vi "NP_IOW_LaunchTheServer.vi"(5 "error in (no error)":errorcluster) -> (19 "error out":errorcluster)   [LabVIEW 2010]
uses:
  <vilib>/registry/registry.llb/Registry View.ctl
  <vilib>/registry/registry.llb/Registry SAM.ctl
  <vilib>/registry/registry.llb/Registry RtKey.ctl
  <vilib>/registry/registry.llb/Read Registry Value Simple STR.vi
panel:
  out "NSTRUCT Instrument Manager path":string
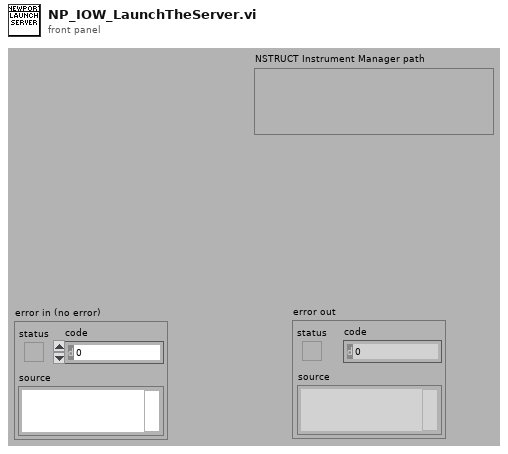
[diagram p1: front panel]
types:
  T1 = typedef "Registry SAM.ctl" = enum32{"KEY_QUERY_VALUE", "KEY_SET_VALUE", "KEY_CREATE_SUB_KEY", "KEY_ENUMERATE_SUB_KEYS", "KEY_NOTIFY", "KEY_CREATE_LINK", "KEY_READ", "KEY_WRITE", "KEY_ALL_ACCESS", "KEY_READ | KEY_WRITE"}
  T2 = typedef "Registry RtKey.ctl" = enum32{"HKEY_CLASSES_ROOT", "HKEY_CURRENT_USER", "HKEY_LOCAL_MACHINE", "HKEY_USERS", "HKEY_PERFORMANCE_DATA", "HKEY_CURRENT_CONFIG", "HKEY_DYN_DATA"}
  T3 = typedef "Registry View.ctl" = u16
  T4 = typedef "Registry refnum.ctl" = refnum<k1>
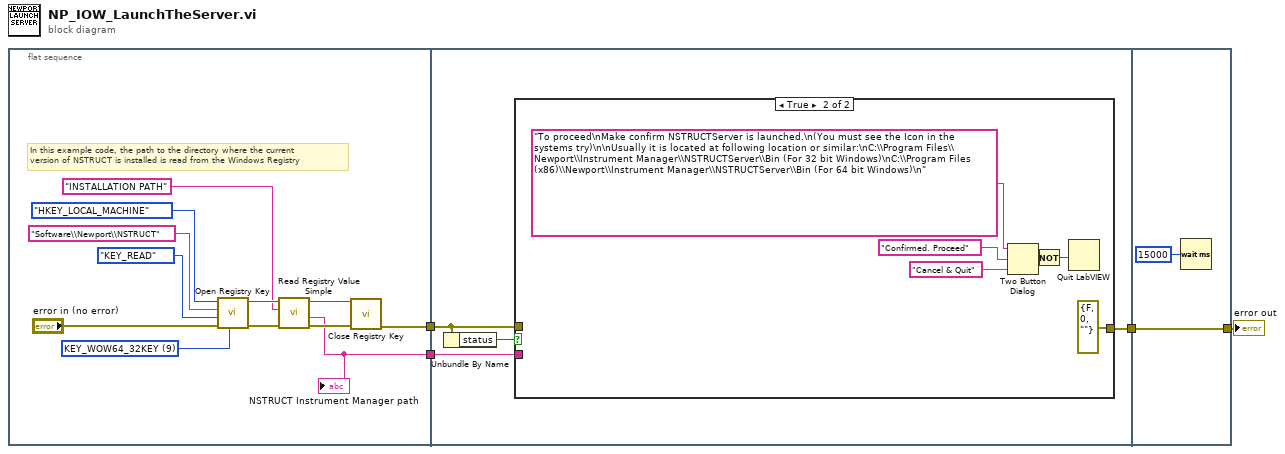
[diagram p0: block diagram]
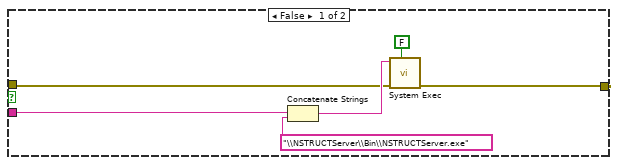
[diagram p2: hidden frame]
diagram:
  n1 = flat-sequence {
    tunnel: [w6] -> w4
    tunnel: [w5] -> w3
    tunnel: w4 -> [w18]
    tunnel: w3 -> [w20]
    tunnel: [w17] -> w1
    tunnel: [w34] -> w2
    tunnel: w1 -> [w34]
    frame #0 {
      w10 = T3 9 items=["Default"=0, "KEY_WOW64_64KEY"=8, "KEY_WOW64_32KEY"=9] ("registry view")
      # "In this example code, the path to the directory where the current\nversion of NSTRUCT is installed is read from the Windows Registry"
      n2 = call <vilib>:"Open Registry Key.vi"("registry view"=w10, "error in (no error)"="error in (no error)", "security access mask (KEY_READ | KEY_WRITE)"=Registry_SAM."KEY_READ", "subkey"="Software\\Newport\\NSTRUCT", "root key (HKEY_LOCAL_MACHINE)"=Registry_RtKey."HKEY_LOCAL_MACHINE") -> ("error out"=w16:errorcluster, "refnum out"=w13:T4)  [unwired: 5 out]
      n3 = call-poly <vilib>:"Read Registry Value Simple.vi"("error in (no error)"=w16, "value"="INSTALLATION PATH" ("default data"), "refnum"=w13) -> ("error out"=w8:errorcluster, "String/Binary data"=w5:string, "refnum out"=w9:T4)  [unwired: 1 in, 3 out]
      "NSTRUCT Instrument Manager path" <- w5
      n4 = call <vilib>:"Close Registry Key.vi"("error in (no error)"=w8, "refnum"=w9) -> ("error out"=w6:errorcluster)  [unwired: 5 out]
    }
    frame #1 {
      n5 = Unbundle By Name(w18) -> ("status"=w19:bool)
      n6 = case shown="True" w19 {
        tunnel: w20 -> [w26 _]
        tunnel: w18 -> [w22 _]
        tunnel: [w21 errorcluster {"status"=FALSE, "code"=0, "source"=""} ("error out")] -> w17
        frame False {
          n7 = Concatenate Strings(w26, "\\NSTRUCTServer\\Bin\\NSTRUCTServer.exe") -> (w24:string)
          n8 = call <vilib>:"System Exec.vi"("wait until completion? (T)"=FALSE, "error in (no error)"=w22, "command line"=w24) -> ("error out"=w21:errorcluster)  [unwired: 5 in, 3 out]
        }
        frame True {
          n9 = Two Button Dialog(message="To proceed\nMake confirm NSTRUCTServer is launched.\n(You must see the Icon in the systems try)\n\nUsually it is located at following location or similar:\nC:\\Program Files\\Newport\\Instrument Manager\\NSTRUCTServer\\Bin (For 32 bit Windows)\nC:\\Program Files (x86)\\Newport\\Instrument Manager\\NSTRUCTServer\\Bin (For 64 bit Windows)\n", 1:"Cancel & Quit" ("T button name (\"OK\")"), 2:"Confirmed. Proceed" ("T button name (\"OK\")")) -> (T button?=w29:bool)
          n10 = Not(x=w29) -> (.not. x?=w28:bool)
          n11 = Quit LabVIEW(quit? (T)=w28) -> ()
        }
      }
    }
    frame #2 {
      n12 = Wait (ms)(milliseconds to wait=u32 15000) -> ()  [unwired: 1 out]
    }
  }
  "error out" <- w2
